vi "LcWebView_example_3.vi"() -> ()   [LabVIEW 2019, in "LcWebView.lvclass"]
doc: "Inject javascript arguments"
uses:
  LcWebView.lvclass
  C:/Projects/WebView2/LcWebView/data/Microsoft.Web.WebView2.WinForms.dll
panel:
  out "BrowserProcessId":u32
  out "Source Change":string
  out "Initialise Loops":i32
  out "Status Message":string
  out "Status":i32(ring) items=["Created", "WaitingForActivation", "WaitingToRun", "Running", "WaitingForChildrenToComplete", "RanToCompletion", "Canceled", "Faulted"]
  in  "stop":bool
  in  "Web":refnum<k24>(container)
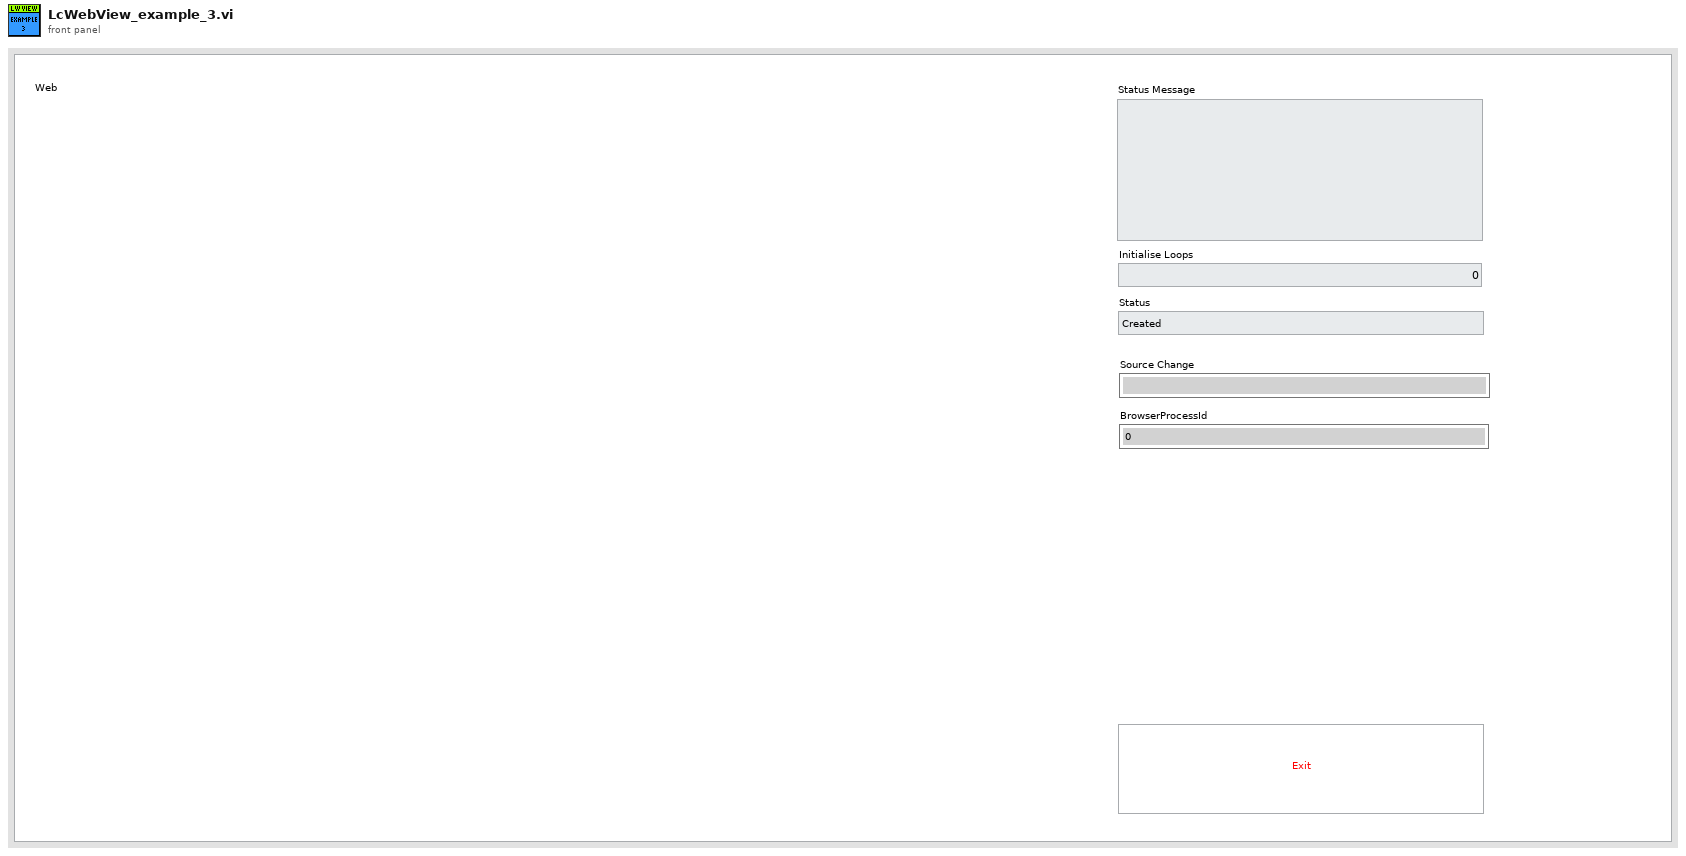
[diagram p1: front panel]
types:
  T1 = typedef "LcWebView.lvclass/WebViewDynamicEvents.ctl" = cluster{"Event Registration Ref":refnum<event-registration>, "Source event":refnum<user-event>}
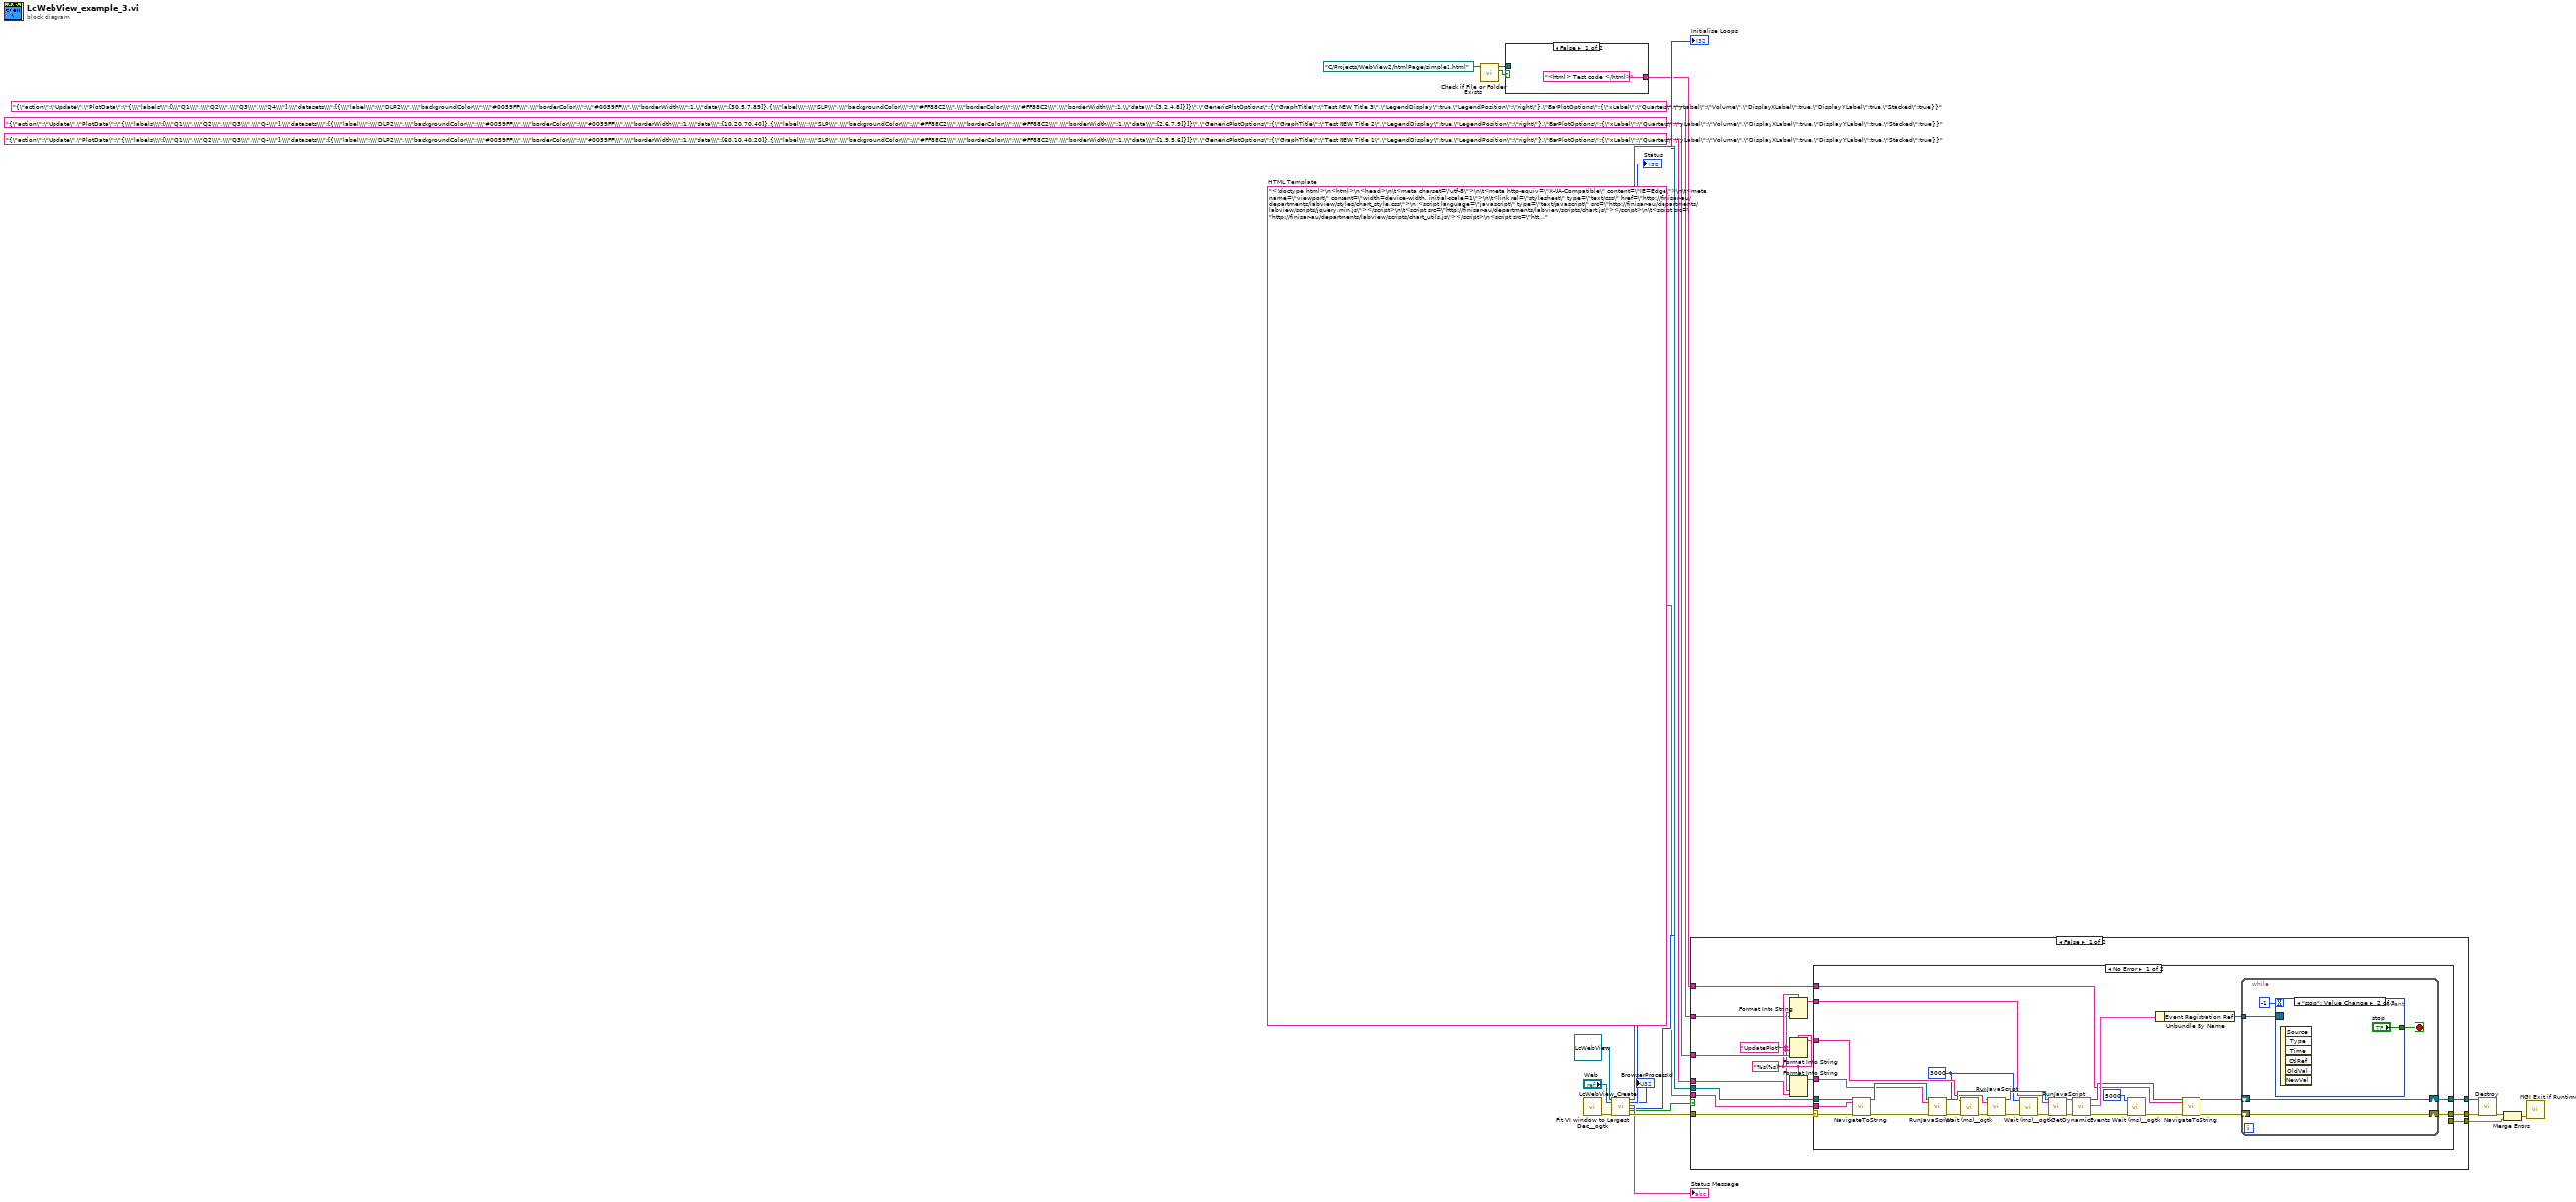
[diagram p0: block diagram]
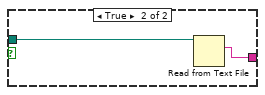
[diagram p2: hidden frame]
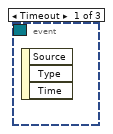
[diagram p3: hidden frame]
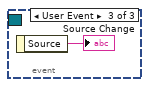
[diagram p4: hidden frame]
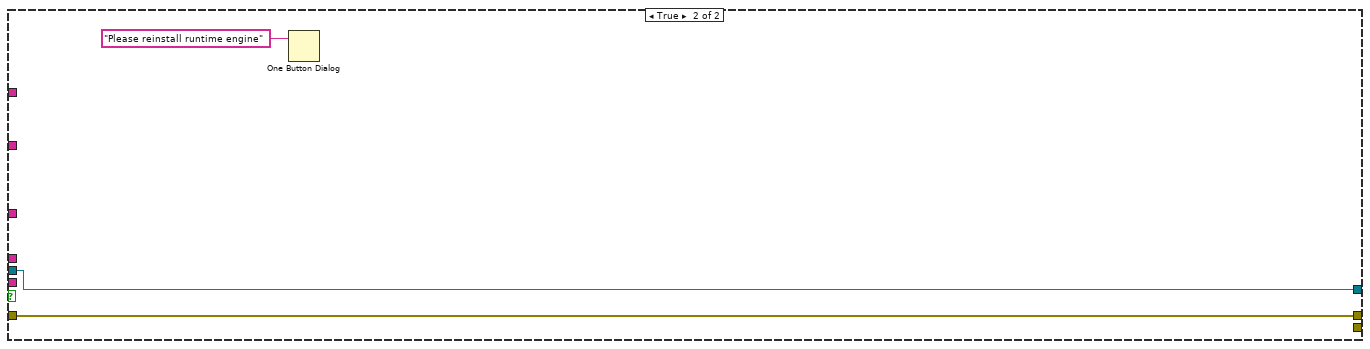
[diagram p6: hidden frame]
diagram:
  w9 = "<!doctype html>\n<html>\n<head>\n\t<meta charset=\"utf-8\">\n\t<meta http-equiv=\"X-UA-Compatible\" content=\"IE=Edge\">\n\t<meta name=\"viewport\" content=\"width=device-width, initial-scale=1\">\n\t<link rel=\"stylesheet\" type=\"text/css\" href=\"http://finisar-au/departments/labview/styles/chart_style.css\">\n <script language=\"javascript\" type=\"text/javascript\" src=\"http://finisar-au/departments/labview/scripts/jquery.min.js\"></script>\n\t<script src=\"http://finisar-au/departments/labview/scripts/chart.js\"></script>\n\t<script src=\"http://finisar-au/departments/labview/scripts/chart_utils.js\"></script>\n<script src=\"http://finisar-au/departments/labview/scripts/json2.js\"></script>\n    <script src=\"http://finisar-au/departments/labview/scripts/jquery(v1.11.3).min.js\"></script>\n    <style>\n    \t#container{\n            width:95vm;\n            height:95vh;\n            }\n        #canvas {\n\t\t-moz-user-select: none;\n\t\t-webkit-user-select: none;\n\t\t-ms-user-select: none;  \n\t   }\n\t    </style>\n</head>\n\n<body>\n<div id=\"container\">\n\t\t<canvas id=\"canvas\"></canvas>\n\t</div>\n\t<script type=\"text/javascript\">\n//---colour helper\nvar color = Chart.helpers.color;\nvar plotData ={}  \n\n // summarise config here --------------------------                   \n        var config = {\n\n// **************** PLOT TYPE***************************\n\t\t\ttype: 'bar',\n\n\t\t\tdata: plotData,\n//\t\t\t **************** PLOT OPTIONS : THIS PART WILL BE PLOT TYPE DEPENDENT***************************\noptions: \n{\nresponsive: true,\nmaintainAspectRatio: false,\n\t\t\t\tanimation: {\n\t\t\t\t\tanimateScale: true,\n\t\t\t\t\tanimateRotate: true\n\t\t\t\t},\nlegend: {\ndisplay:false,\t\t\t\t\t\t\nposition: 'right'\n\t\t\t\t\t},\ntitle: {\n\t\t\t\t\t\tdisplay:true,\n\t\t\t\t\t\ttext: 'INPUT'\n\t\t\t\t\t},  \n//*************************  ADDITIONAL OPTIONS   ***********************\n\t\t\t\tscales: {\n\t\t\t\t\txAxes: [{\n\t\t\t\t\t\t\tscaleLabel: {\n\t\t\t\t\t\t\tdisplay: true,\n\t\t\t\t\t\t\tlabelString: 'INPUT',\n       stacked:true\n\t\t\t\t\t\t}\n\t\t\t\t\t}],\n\t\t\t\t\tyAxes: [{\n\tticks: {\n\t\t\t\t\t\t\tmin: 0\n\t\t\t\t\t\t\t\t\t\t\t\t\t},\n\t\t\t\t\t\tscaleLabel: {\n\t\t\t\t\t\t\tdisplay: true,\n\t\t\t\t\t\t\tlabelString: 'INPUT',\n       stacked:true\n       \t\t\t\t\t\t}\n\t\t\t\t\t}]\n\t\t\t\t},\ntooltips: {\nenabled: true}\t\n}\n\t\t};\n\n// run plot function here -------------------------- \nwindow.onload = function() {\n\t  var ctx = document.getElementById('canvas').getContext('2d');\n\t\t\twindow.myChart = new Chart(ctx, config); \n};\n\nfunction UpdatePlot(data) {        \n    var myData = JSON.parse(data.PlotData);\n    config.data=myData;\n\tconfig.options.legend.display= data.GenericPlotOptions.LegendDisplay;\n\tconfig.options.legend.position=data.GenericPlotOptions.LegendPosition;            \n\tconfig.options.title.text=data.GenericPlotOptions.GraphTitle;\n\n//*************************  ADDITIONAL OPTIONS UPDATE ***********************\n\tconfig.options.scales.yAxes[0].stacked=data.BarPlotOptions.Stacked;\n\tconfig.options.scales.xAxes[0].stacked=data.BarPlotOptions.Stacked;\n\tconfig.options.scales.xAxes[0].scaleLabel.labelString=data.BarPlotOptions.xLabel;\n\tconfig.options.scales.yAxes[0].scaleLabel.labelString=data.BarPlotOptions.yLabel;\n\tconfig.options.scales.yAxes[0].scaleLabel.display=data.BarPlotOptions.DisplayYLabel;\n\tconfig.options.scales.xAxes[0].scaleLabel.display=data.BarPlotOptions.DisplayXLabel;\n\n//*************************  UPDATE PLOT ***********************\n\twindow.myChart.update();\n}\n\t</script>\n</body>\n</html>"  # HTML Template
  n1 = call <vilib>:"Check if File or Folder Exists.vi"("path"=path "C:/Projects/WebView2/htmlPage/simple1.html" ("DLLs path In")) -> ("file or folder exists?"=w5:bool, "dup path"=w4:path)  [unwired: 8 in, 1 out]
  n2 = case shown="False" w5 {
    tunnel: w4 -> [_ w26]
    tunnel: ["<html> Test code </html>" ("HTML Content") w25] -> w2
    frame False {
    }
    frame True {
      n3 = Read from Text File(file (use dialog)=w26) -> (text=w25:string)  [unwired: 3 in, 3 out]
    }
  }
  n4 = call "Fit VI window to Largest Dec__ogtk.vi"() -> ("error out"=w11:errorcluster)  [unwired: 6 in, 1 out]
  n5 = call "LcWebView_Create.vi"("reference in"=refnum<class "LcWebView.lvclass"> refnum, "Webview container"="Web", "Error In"=w11) -> ("BrowserProcessId"=→"BrowserProcessId":u32, "reference out"=w21:refnum<class "LcWebView.lvclass">, "Status"=→"Status":i32, "Status Message"=→"Status Message":string, "Initialise Loops"=→"Initialise Loops":i32, "Reinstall Runtime"=w12:bool, "Error Out"=w20:errorcluster)  [unwired: 9 in, 1 out]
  n6 = case shown="False" w12 {
    tunnel: w21 -> [w41 w81]
    tunnel: w20 -> [w40 w80]
    tunnel: [w39 w81] -> w19
    tunnel: [w38 w80] -> w18
    tunnel: [w37 _] -> w13
    tunnel: w9 -> [w36 _]
    tunnel: "{\"action\":\"Update\",\"PlotData\":\"{\\\"labels\\\":[\\\"Q1\\\",\\\"Q2\\\",\\\"Q3\\\",\\\"Q4\\\"],\\\"datasets\\\":[{\\\"label\\\":\\\"DLP2\\\",\\\"backgroundColor\\\":\\\"#0059FF\\\",\\\"borderColor\\\":\\\"#0059FF\\\",\\\"borderWidth\\\":1,\\\"data\\\":[60,10,40,20]},{\\\"label\\\":\\\"SLP\\\",\\\"backgroundColor\\\":\\\"#FF88C2\\\",\\\"borderColor\\\":\\\"#FF88C2\\\",\\\"borderWidth\\\":1,\\\"data\\\":[1,9,5,6]}]}\",\"GenericPlotOptions\":{\"GraphTitle\":\"Test NEW Title 1\",\"LegendDisplay\":true,\"LegendPosition\":\"right\"},\"BarPlotOptions\":{\"xLabel\":\"Quarters\",\"yLabel\":\"Volume\",\"DisplayXLabel\":true,\"DisplayYLabel\":true,\"Stacked\":true}}" ("Java Script Function") -> [w35 _]
    tunnel: "{\"action\":\"Update\",\"PlotData\":\"{\\\"labels\\\":[\\\"Q1\\\",\\\"Q2\\\",\\\"Q3\\\",\\\"Q4\\\"],\\\"datasets\\\":[{\\\"label\\\":\\\"DLP2\\\",\\\"backgroundColor\\\":\\\"#0059FF\\\",\\\"borderColor\\\":\\\"#0059FF\\\",\\\"borderWidth\\\":1,\\\"data\\\":[10,20,70,40]},{\\\"label\\\":\\\"SLP\\\",\\\"backgroundColor\\\":\\\"#FF88C2\\\",\\\"borderColor\\\":\\\"#FF88C2\\\",\\\"borderWidth\\\":1,\\\"data\\\":[2,6,7,9]}]}\",\"GenericPlotOptions\":{\"GraphTitle\":\"Test NEW Title 2\",\"LegendDisplay\":true,\"LegendPosition\":\"right\"},\"BarPlotOptions\":{\"xLabel\":\"Quarters\",\"yLabel\":\"Volume\",\"DisplayXLabel\":true,\"DisplayYLabel\":true,\"Stacked\":true}}" ("Java Script Function") -> [w33 _]
    tunnel: "{\"action\":\"Update\",\"PlotData\":\"{\\\"labels\\\":[\\\"Q1\\\",\\\"Q2\\\",\\\"Q3\\\",\\\"Q4\\\"],\\\"datasets\\\":[{\\\"label\\\":\\\"DLP2\\\",\\\"backgroundColor\\\":\\\"#0059FF\\\",\\\"borderColor\\\":\\\"#0059FF\\\",\\\"borderWidth\\\":1,\\\"data\\\":[30,5,7,89]},{\\\"label\\\":\\\"SLP\\\",\\\"backgroundColor\\\":\\\"#FF88C2\\\",\\\"borderColor\\\":\\\"#FF88C2\\\",\\\"borderWidth\\\":1,\\\"data\\\":[3,2,4,8]}]}\",\"GenericPlotOptions\":{\"GraphTitle\":\"Test NEW Title 3\",\"LegendDisplay\":true,\"LegendPosition\":\"right\"},\"BarPlotOptions\":{\"xLabel\":\"Quarters\",\"yLabel\":\"Volume\",\"DisplayXLabel\":true,\"DisplayYLabel\":true,\"Stacked\":true}}" ("Java Script Function") -> [w30 _]
    tunnel: w2 -> [w27 _]
    frame False {
      w31 = "UpdatePlot" ("input 1")
      w32 = "%s(%s)" ("format string")
      n7 = Format Into String(format string=w32, w31, w30) -> (resulting string=w28:string)  [unwired: 2 in, 1 out]
      n8 = Format Into String(format string=w32, w31, w33) -> (resulting string=w29:string)  [unwired: 2 in, 1 out]
      n9 = Format Into String(format string=w32, w31, w35) -> (resulting string=w34:string)  [unwired: 2 in, 1 out]
      n10 = case shown="No Error" w40 {
        selector: w40 -> [w66 w77]
        tunnel: w41 -> [w67 w78]
        tunnel: [w69 w78] -> w39
        tunnel: [w68 _] -> w38
        tunnel: [_ w77] -> w37
        tunnel: w36 -> [w65 _]
        tunnel: w34 -> [w63 _]
        tunnel: w29 -> [w56 _]
        tunnel: w28 -> [w55 _]
        tunnel: w27 -> [w43 _]
        frame No Error {
          w54 = u32 3000 ("milliseconds to wait")
          n11 = call-dynamic "NavigateToString.vi"("reference in"=w67, "HTML Content"=w65, "Error In"=w66) -> ("reference out"=w64:refnum<class "LcWebView.lvclass">, "Error Out"=w42:errorcluster)  [unwired: 14 in, 1 out]
          n12 = call-dynamic "RunJavaScript.vi"("reference in"=w64, "Java Script Function"=w63, "Error In"=w42) -> ("reference out"=w62:refnum<class "LcWebView.lvclass">, "Error Out"=w60:errorcluster)  [unwired: 13 in, 2 out]
          n13 = call "Wait (ms)__ogtk.vi"("error in (no error)"=w60, "milliseconds to wait"=w54) -> ("error out"=w59:errorcluster)  [unwired: 8 in, 1 out]
          n14 = call-dynamic "RunJavaScript.vi"("reference in"=w62, "Java Script Function"=w56, "Error In"=w59) -> ("reference out"=w61:refnum<class "LcWebView.lvclass">, "Error Out"=w58:errorcluster)  [unwired: 13 in, 2 out]
          n15 = call "Wait (ms)__ogtk.vi"("error in (no error)"=w58, "milliseconds to wait"=w54) -> ("error out"=w57:errorcluster)  [unwired: 8 in, 1 out]
          n16 = call-dynamic "RunJavaScript.vi"("reference in"=w61, "Java Script Function"=w55, "Error In"=w57) -> ("reference out"=w53:refnum<class "LcWebView.lvclass">, "Error Out"=w52:errorcluster)  [unwired: 13 in, 2 out]
          n17 = call-dynamic "GetDynamicEvents.vi"("reference in"=w53, "Error In"=w52) -> ("reference out"=w49:refnum<class "LcWebView.lvclass">, "DynamicEvents"=w51:T1, "Error Out"=w45:errorcluster)  [unwired: 15 in]
          n18 = call "Wait (ms)__ogtk.vi"("error in (no error)"=w45, "milliseconds to wait"=u32 5000) -> ("error out"=w46:errorcluster)  [unwired: 8 in, 1 out]
          n19 = Unbundle By Name(w51) -> ("Event Registration Ref"=w50:refnum<event-registration>)
          n20 = call-dynamic "NavigateToString.vi"("reference in"=w49, "HTML Content"=w43, "Error In"=w46) -> ("reference out"=w48:refnum<class "LcWebView.lvclass">, "Error Out"=w47:errorcluster)  [unwired: 14 in, 1 out]
          n21 = while {
            shift-right: [w74] -> w69
            shift-left: w48 -> [w74]
            shift-right: [w73] -> w68
            shift-left: w47 -> [w73]
            tunnel: w50 -> [w72]
            stop <- w70 stop-if-true
            n22 = event shown="[1] \"stop\": Value Change" {
              selector: w72 -> [_ _ _]
              dyn-events: _ -> [_ _ _]
              timeout: -1 -> [_ _ _]
              tunnel: [_ "stop" _] -> w70
              event Timeout {
                n23 = event-data() -> ()  [unwired: 1 in, 3 out]
              }
              event "stop": Value Change {
                n24 = event-data() -> ()  [unwired: 1 in, 6 out]
              }
              event User Event {
                n25 = event-data() -> ("Source"=→"Source Change":string)  [unwired: 1 in]
              }
            }
          }
        }
        frame Error {
        }
      }
    }
    frame True {
      n26 = One Button Dialog(message="Please reinstall runtime engine") -> ()  [unwired: 1 in, 1 out]
    }
  }
  n27 = call-dynamic "Destroy.vi"("reference in"=w19, "Error In"=w18) -> ("Error Out"=w17:errorcluster)  [unwired: 16 in, 1 out]
  n28 = Merge Errors(w17, w13) -> (w10:errorcluster)
  n29 = call "MGI Exit if Runtime.vi"("Error In (Dependency Only)"=w10) -> ()  [unwired: 11 in]
